vi "main.vi"() -> ()   [LabVIEW 2014]
uses:
  <vilib>/httpClient/POSTBuffer.vi
  <vilib>/httpClient/LabVIEWHTTPClient.lvlib
panel:
  out "body":string
  out "headers":string
  out "Waveform Graph":dbl[](graph)
  out "Array num":dbl[](array[numeric])
  out "Array string":string[](array[string])
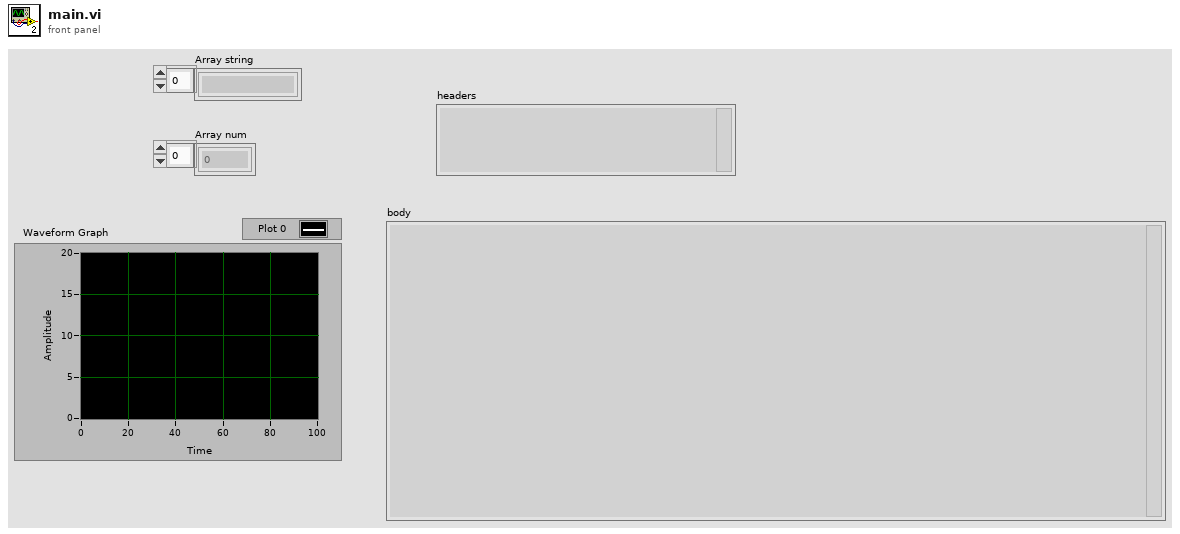
[diagram p1: front panel]
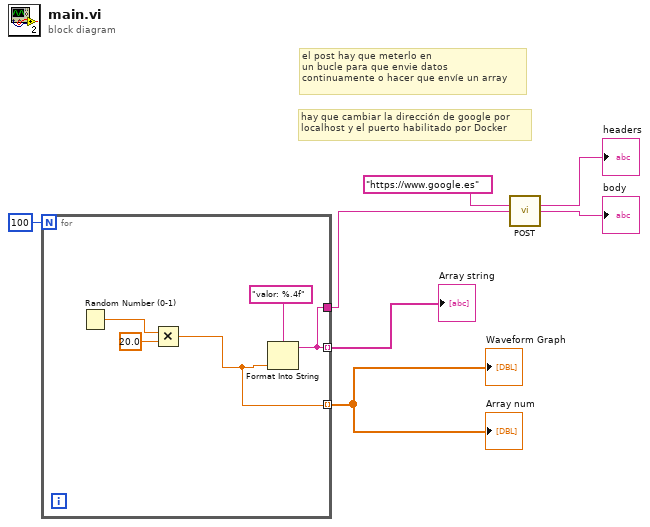
[diagram p0: block diagram]
diagram:
  # "hay que cambiar la dirección de google por\nlocalhost y el puerto habilitado por Docker"
  # "el post hay que meterlo en\nun bucle para que envie datos\ncontinuamente o hacer que envíe un array"
  n1 = for {
    N: 100 -> [_]
    tunnel: [w8] -> w5 mode=indexing
    tunnel: [w9] -> w4 mode=indexing
    tunnel: [w8] -> w3
    n2 = Random Number (0-1)() -> (number: 0 to 1=w12:dbl)
    n3 = Multiply(x=w12, y=20.0) -> (x*y=w9:dbl)
    n4 = Format Into String(format string="valor: %.4f", w9) -> (resulting string=w8:string)  [unwired: 2 in, 1 out]
  }
  "Array string" <- w5
  "Array num" <- w4
  "Waveform Graph" <- w4
  n5 = call-poly <vilib>:"POST.vi"("url"="https://www.google.es", "buffer"=w3) -> ("headers"=→"headers":string, "body"=→"body":string)  [unwired: 10 in, 2 out]
